vi "MapResult Create.vi"(8 "error in (no error)":errorcluster, 10 "InsertResultVariant":variant, 11 "DbConnection in":refnum<class "DbConnection.lvclass">) -> (0 "error out":errorcluster, 2 "ID":variant)   [LabVIEW 2020, in "ORM.lvlib" / "DbConnection.lvclass"]
uses:
  DbConnection.lvclass
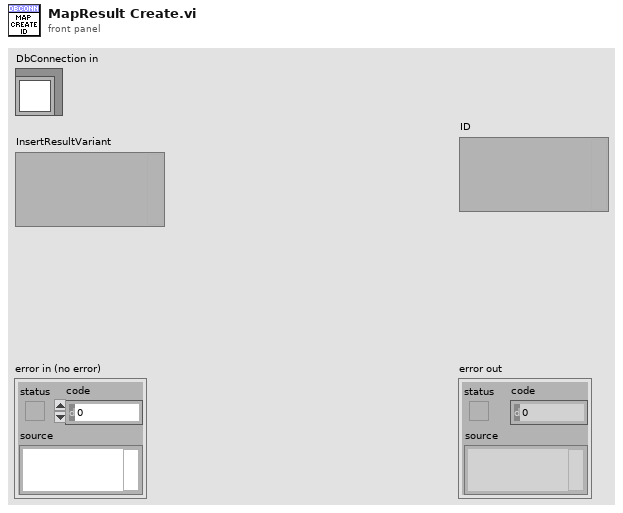
[diagram p1: front panel]
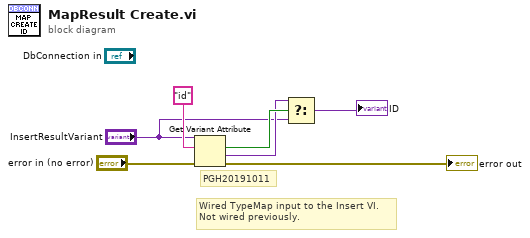
[diagram p0: block diagram]
diagram:
  # "Wired TypeMap input to the Insert VI.\nNot wired previously."
  # "PGH20191011"
  n1 = Get Variant Attribute(Variant="InsertResultVariant", name="id", error in="error in (no error)") -> (found=w6:bool, value=w5:variant, error out=→"error out":errorcluster)  [unwired: 1 in, 1 out]
  n2 = Select(t=w5, s=w6, f="InsertResultVariant") -> (s? t:f=→"ID":variant)
